vi "地址索引编码.vi"(8 "error in (no error)":errorcluster, 9 "简易流程Id":u16, 10 "是否是简易流程":bool, 11 "参数簇":T1={"启动参数"=1, "启动模式"=enum."跨度核查", "量程"=enum."低量程"} {"启动参数" items=["总磷"=1, "总氮"=2, "氨氮"=3]}) -> (0 "error out":errorcluster, 2 "数组":u16[](array[numeric]))   [LabVIEW 2016, in "斯坦道氨氮.lvlib"]
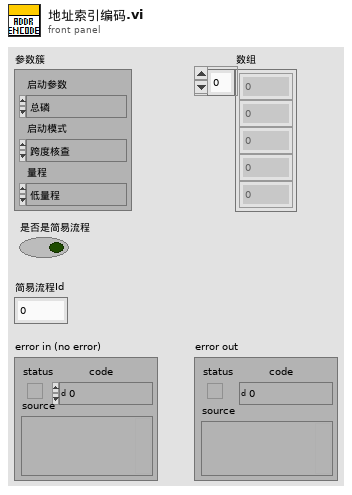
[diagram p1: front panel]
types:
  T1 = cluster{"启动参数":u16, "启动模式":enum16{"跨度核查", "水样测量", "零点核查", "标样核查", "加标回收", "平行样测试", "空白校准", "标样校准", "空白测试"}, "量程":enum16{"低量程", "高量程"}}
  T2 = enum16{"跨度核查", "水样测量", "零点核查", "标样核查", "加标回收", "平行样测试", "空白校准", "标样校准", "空白测试"}
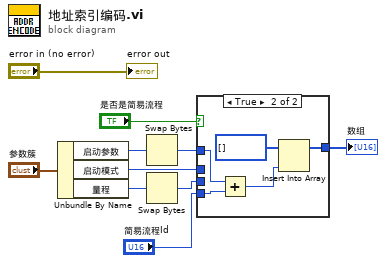
[diagram p0: block diagram]
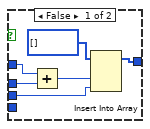
[diagram p2: hidden frame]
diagram:
  n1 = Unbundle By Name("参数簇") -> ("启动参数"=w4:u16, "启动模式"=w3:T2, "量程"=w2:enum16{"低量程", "高量程"})
  n2 = Swap Bytes(anything=w4) -> (byte swapped=w6:u16)
  n3 = Swap Bytes(anything=w2) -> (byte swapped=w7:u16)
  n4 = case shown="True" "是否是简易流程" {
    tunnel: [w14 w19] -> w8
    tunnel: w3 -> [w13 _]
    tunnel: w6 -> [w12 w18]
    tunnel: w7 -> [w11 _]
    tunnel: "简易流程Id" -> [_ w17]
    frame False {
      n5 = Add(x=w12, y=w13) -> (x+y=w16:u16)
      n6 = Insert Into Array(array=u16[] [] ("数组"), new element #1=w16, new element #2=w11) -> (w14:u16[])  [unwired: 1 in]
    }
    frame True {
      n7 = Add(x=w18, y=w17) -> (x+y=w21:u16)
      n8 = Insert Into Array(array=u16[] [] ("数组"), new element=w21) -> (w19:u16[])  [unwired: 1 in]
    }
  }
  "数组" <- w8
  "error out" <- "error in (no error)"
